vi "obtain_data_queue.vi"(8 "error in (no error)":errorcluster, 11 "GenericToplevelComponent in":refnum<class "GenericToplevelComponent.lvclass">) -> (0 "error out":errorcluster, 2 "data queue":refnum<queue>, 3 "GenericToplevelComponent out":refnum<class "GenericToplevelComponent.lvclass">)   [LabVIEW 2010, in "GenericToplevelComponent.lvclass"]
uses:
  GenericToplevelComponent.lvclass
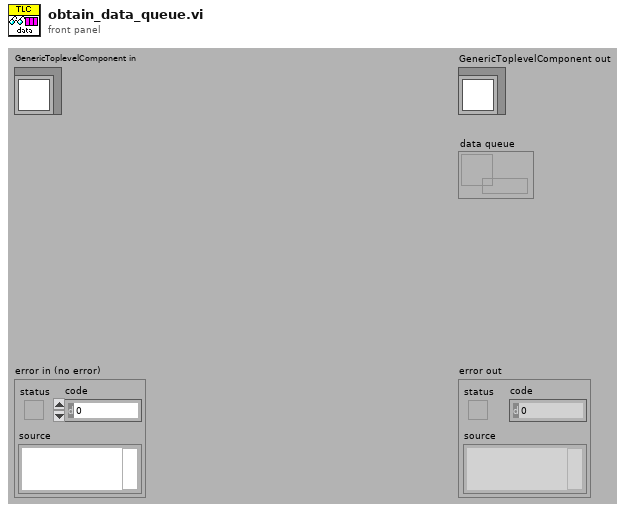
[diagram p1: front panel]
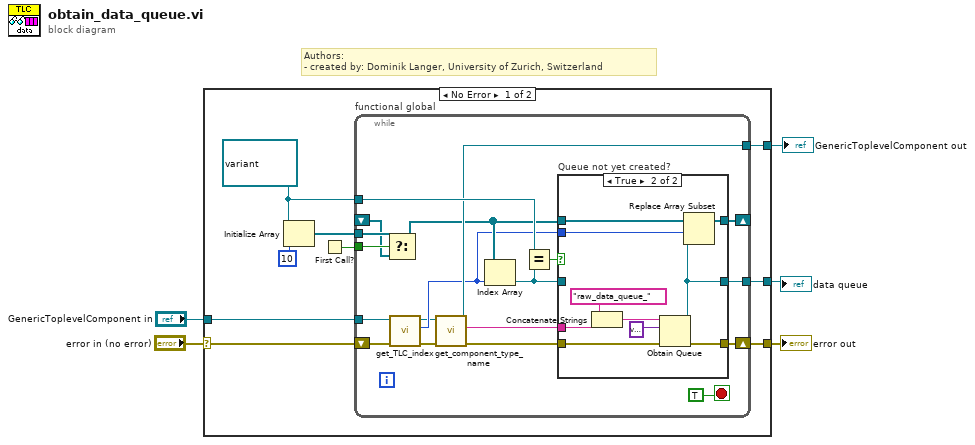
[diagram p0: block diagram]
diagram:
  # "Authors: \n- created by: Dominik Langer, University of Zurich, Switzerland"
  n1 = case shown="No Error" "error in (no error)" {
    selector: "error in (no error)" -> [w9 w48]
    tunnel: [w13 w47] -> w1
    tunnel: "GenericToplevelComponent in" -> [w12 w47]
    tunnel: [w11 _] -> w2
    tunnel: [w10 w48] -> w3
    frame No Error {
      w8 = refnum<queue> refnum ("queue out")
      n2 = Initialize Array(w8, 10 ("dimension size")) -> (w7:refnum<queue>[])
      n3 = First Call?() -> (First Call?: T/F=w6:bool)
      n4 = while "functional global" {
        shift-right: [w31] -> _
        shift-left: _ -> [w21]
        shift-right: [w30] -> w10
        shift-left: w9 -> [w16]
        tunnel: [w27] -> w11
        tunnel: w8 -> [w26]
        tunnel: [w25] -> w13
        tunnel: w12 -> [w18]
        tunnel: w7 -> [w23]
        tunnel: w6 -> [w24]
        stop <- TRUE stop-if-true
        n5 = Select(t=w23, s=w24, f=w21) -> (s? t:f=w22:refnum<queue>[])
        n6 = call "get_TLC_index.vi"("error in (no error)"=w16, "GenericToplevelComponent in"=w18) -> ("error out"=w15:errorcluster, "index"=w19:i32, "GenericToplevelComponent out"=w17:refnum<class "GenericToplevelComponent.lvclass">)  [unwired: 7 in]
        n7 = call-dynamic "get_component_type_name.vi"("error in (no error)"=w15, "GenericPlugin in"=w17) -> ("error out"=w20:errorcluster, "component type"=w33:string, "GenericPlugin out"=w25:refnum<class "GenericToplevelComponent.lvclass">)  [unwired: 7 in]
        n8 = Index Array(array=w22, index=w19) -> (element=w28:refnum<queue>)
        n9 = Equal?(x=w26, y=w28) -> (x = y?=w32:bool)
        n10 = case "Queue not yet created?" shown="True" w32 {
          tunnel: w20 -> [w36 w44]
          tunnel: w33 -> [_ w43]
          tunnel: [w36 w42] -> w30
          tunnel: w22 -> [w35 w41]
          tunnel: [w35 w38] -> w31
          tunnel: w28 -> [w34 _]
          tunnel: [w34 w39] -> w27
          tunnel: w19 -> [_ w40]
          frame False {
          }
          frame True {
            n11 = Concatenate Strings("raw_data_queue_" ("string"), w43) -> (w46:string)
            n12 = Obtain Queue(name (unnamed)=w46, element data type=variant ("variant"), error in (no error)=w44) -> (queue out=w39:refnum<queue>, error out=w42:errorcluster)  [unwired: 2 in, 1 out]
            n13 = Replace Array Subset(array=w41, new element=w39, index=w40) -> (w38:refnum<queue>[])
          }
        }
      }
    }
    frame Error {
    }
  }
  "error out" <- w3
  "GenericToplevelComponent out" <- w1
  "data queue" <- w2
